vi "flushAllQueuesAndFIFOs.vi"(8 "error in (no error)":errorcluster, 10 "Queues":T1, 11 "FPGA VI ref":T2) -> (0 "error out":errorcluster)   [LabVIEW 2010]
uses:
  FPGA_ref.ctl
  internal_queues.ctl
  line_info.ctl
  volume_with_lines.ctl
  volume_info.ctl
  kalman_result_scaled.ctl
  location3D.ctl
  <vilib>/rvi/interface/nirviMethod/nirviMethod.xnode
  <vilib>/rvi/interface/common/niFpgaNodeNameForErrorReporting.ctl
  <vilib>/rvi/errors/niLvFpgaWhatHappensToTopLevelVI.ctl
  <vilib>/Utility/error.llb/Error Cluster From Error Code.vi
  <vilib>/rvi/errors/niLvFpgaAdjustHostInterfaceError.vi
  NiFpgaLv.dll
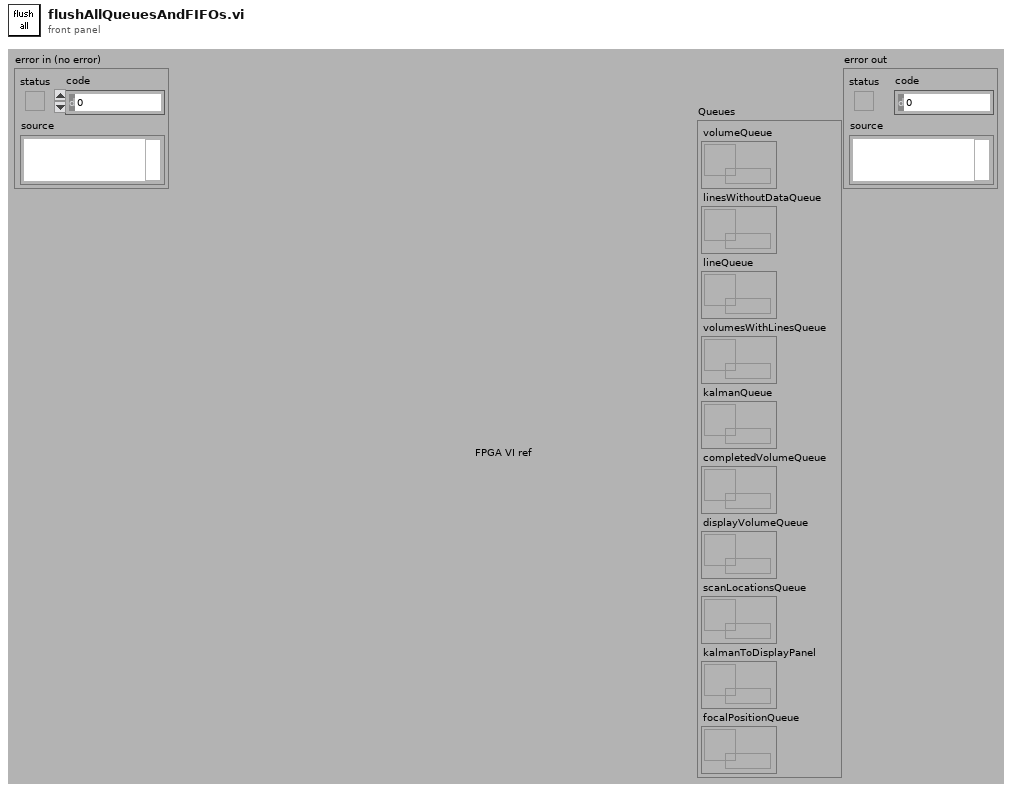
[diagram p1: front panel]
types:
  T1 = typedef "internal_queues.ctl" = cluster{"volumeQueue":refnum<queue>, "linesWithoutDataQueue":refnum<queue>, "lineQueue":refnum<queue>, "volumesWithLinesQueue":refnum<queue>, "kalmanQueue":refnum<queue>, "completedVolumeQueue":refnum<queue>, "displayVolumeQueue":refnum<queue>, "scanLocationsQueue":refnum<queue>, "kalmanToDisplayPanel":refnum<queue>, "focalPositionQueue":refnum<queue>}
  T2 = typedef "FPGA_ref.ctl" = refnum<k20>
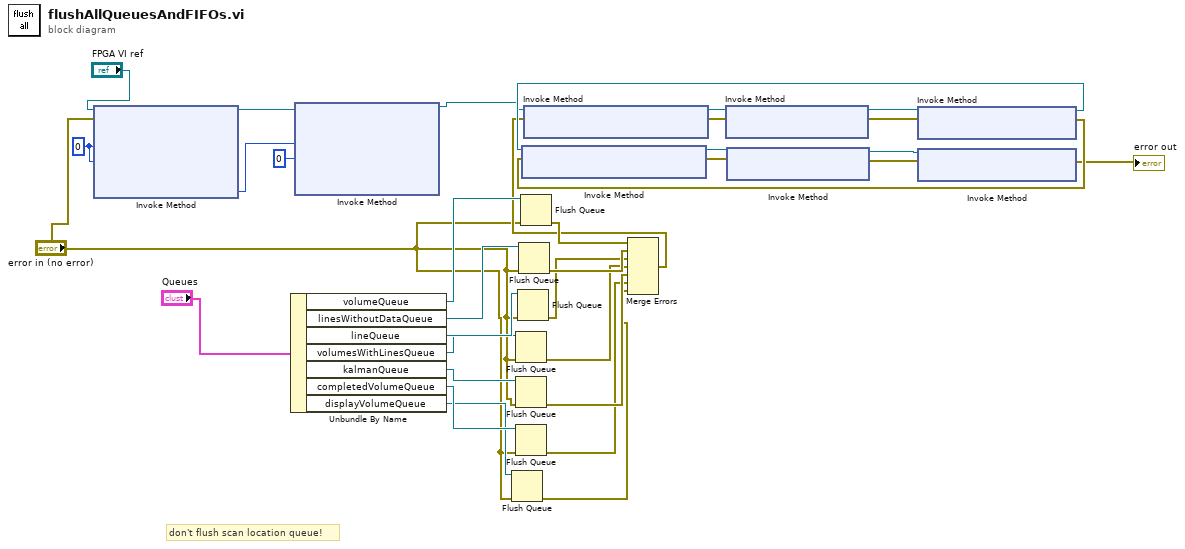
[diagram p0: block diagram]
diagram:
  w6 = u32 0 ("Number of Elements")
  # "don't flush scan location queue!"
  n1 = xnode "Invoke Method"("FPGA VI Reference In"="FPGA VI ref", "error in"="error in (no error)", "Number of Elements"=w6, "Timeout (ms)"=w6) -> ("FPGA VI Reference Out"=w4:T2, "Elements Remaining"=w3:u32)  [unwired: 2 out]
  n2 = Unbundle By Name("Queues") -> ("volumeQueue"=w33:refnum<queue>, "linesWithoutDataQueue"=w32:refnum<queue>, "lineQueue"=w31:refnum<queue>, "volumesWithLinesQueue"=w30:refnum<queue>, "kalmanQueue"=w29:refnum<queue>, "completedVolumeQueue"=w28:refnum<queue>, "displayVolumeQueue"=w27:refnum<queue>)
  n3 = xnode "Invoke Method"("FPGA VI Reference In"=w4, "Number of Elements"=w3, "Timeout (ms)"=0) -> ("FPGA VI Reference Out"=w1:T2)  [unwired: 1 in, 3 out]
  n4 = Flush Queue(queue=w27, error in (no error)="error in (no error)") -> (error out=w20:errorcluster)  [unwired: 2 out]
  n5 = Flush Queue(queue=w30, error in (no error)="error in (no error)") -> (error out=w23:errorcluster)  [unwired: 2 out]
  n6 = Flush Queue(queue=w29, error in (no error)="error in (no error)") -> (error out=w22:errorcluster)  [unwired: 2 out]
  n7 = Flush Queue(queue=w28, error in (no error)="error in (no error)") -> (error out=w21:errorcluster)  [unwired: 2 out]
  n8 = Flush Queue(queue=w31, error in (no error)="error in (no error)") -> (error out=w24:errorcluster)  [unwired: 2 out]
  n9 = Flush Queue(queue=w32, error in (no error)="error in (no error)") -> (error out=w25:errorcluster)  [unwired: 2 out]
  n10 = Flush Queue(queue=w33, error in (no error)="error in (no error)") -> (error out=w26:errorcluster)  [unwired: 2 out]
  n11 = Merge Errors(w26, w25, w24, w23, w22, w21, w20) -> (w9:errorcluster)
  n12 = xnode "Invoke Method"("FPGA VI Reference In"=w1, "error in"=w9) -> ("FPGA VI Reference Out"=w19:T2, "error out"=w13:errorcluster)
  n13 = xnode "Invoke Method"("FPGA VI Reference In"=w19, "error in"=w13) -> ("FPGA VI Reference Out"=w18:T2, "error out"=w12:errorcluster)
  n14 = xnode "Invoke Method"("FPGA VI Reference In"=w18, "error in"=w12) -> ("FPGA VI Reference Out"=w14:T2, "error out"=w15:errorcluster)
  n15 = xnode "Invoke Method"("FPGA VI Reference In"=w14, "error in"=w15) -> ("FPGA VI Reference Out"=w17:T2, "error out"=w11:errorcluster)
  n16 = xnode "Invoke Method"("FPGA VI Reference In"=w17, "error in"=w11) -> ("FPGA VI Reference Out"=w16:T2, "error out"=w10:errorcluster)
  n17 = xnode "Invoke Method"("FPGA VI Reference In"=w16, "error in"=w10) -> ("error out"=→"error out":errorcluster)  [unwired: 1 out]
